vi "Import Export - Create Temp SDFs.vi"(8 "Error In":errorcluster, 11 "Item Ref in":T1 format="%.0x") -> (0 "Error Out":errorcluster, 2 "Temp SDF CD":T1 format="%.0x", 3 "Item Ref out":T1 format="%.0x")   [LabVIEW 2017, in "Scan Engine Custom Device.lvlib"]
uses:
  Scan Engine Custom Device.lvlib
  <vilib>/NI Veristand/Custom Device API/Custom Device Item Ref.ctl
  NationalInstruments.VeriStand.SystemStorage
  <vilib>/NI Veristand/Custom Device API/Custom Device API.lvlib
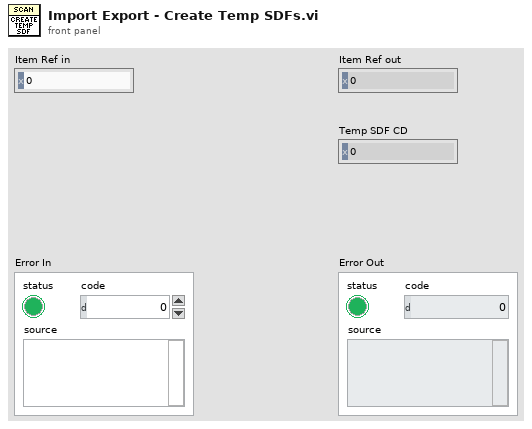
[diagram p1: front panel]
types:
  T1 = typedef "Custom Device API.lvlib/Custom Device Item Ref.ctl" = u64
  T2 = typedef "Custom Device API.lvlib/Custom Device Pointer.ctl" = refnum<k24>
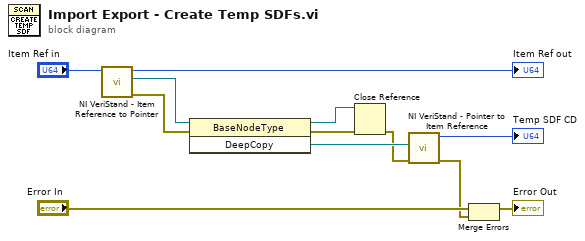
[diagram p0: block diagram]
diagram:
  n1 = call <vilib>:"NI VeriStand - Item Reference to Pointer.vi"("Item Ref in"="Item Ref in") -> ("error out"=w5:errorcluster, "Node Pointer"=w6:T2, "Item Ref out"=→"Item Ref out":T1)  [unwired: 7 in, 1 out]
  n2 = invoke class="BaseNodeType" method="DeepCopy"(reference=w6, error in=w5) -> (reference out=w8:T2, error out=w7:errorcluster, "DeepCopy"=w4:refnum<k24>)  [unwired: 1 in]
  n3 = Close Reference(reference=w8, error in (no error)=w7) -> (error out=w2:errorcluster)
  n4 = call <vilib>:"NI VeriStand - Pointer to Item Reference.vi"("error in (no error)"=w2, "Node Pointer"=w4) -> ("error out"=w1:errorcluster, "Item Ref out"=→"Temp SDF CD":T1)  [unwired: 8 in]
  n5 = Merge Errors("Error In", w1) -> (→"Error Out":errorcluster)
